vi "Distance Calc.vi"() -> ()   [LabVIEW 2014]
panel:
  out "Reference Distance \nin Inches":dbl
  out "Inch per \npixel Value":dbl
  out "Max Distance (Inches)":dbl
  out "Max Pixel Height":dbl
  out "Final Distance Array":dbl[](array[numeric])
  out "CM Heights Array":dbl[](array[numeric])
  in  "Particle Points":dbl[][](array[numeric])
  # "CM(X), CM(Y), Left X, Right X"
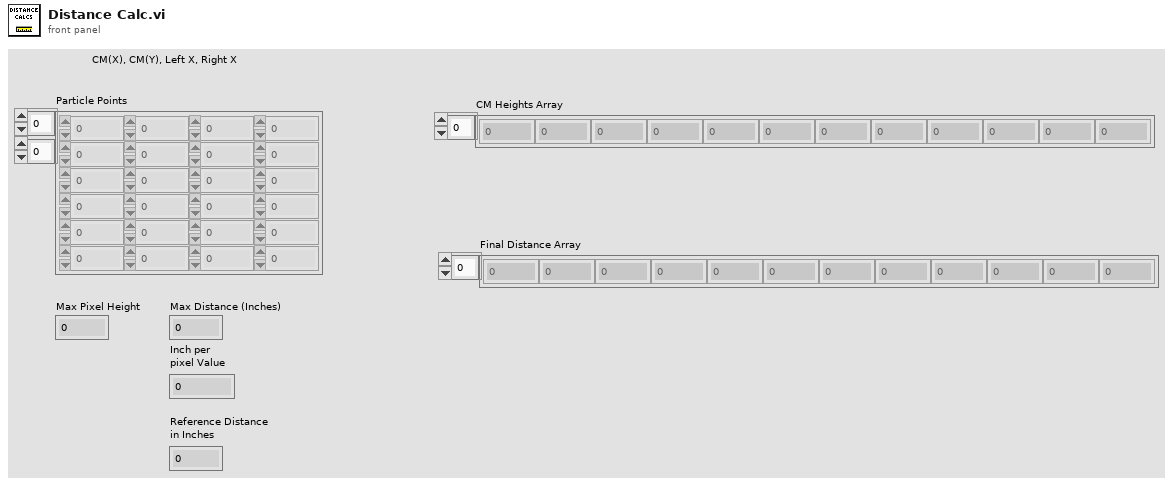
[diagram p1: front panel]
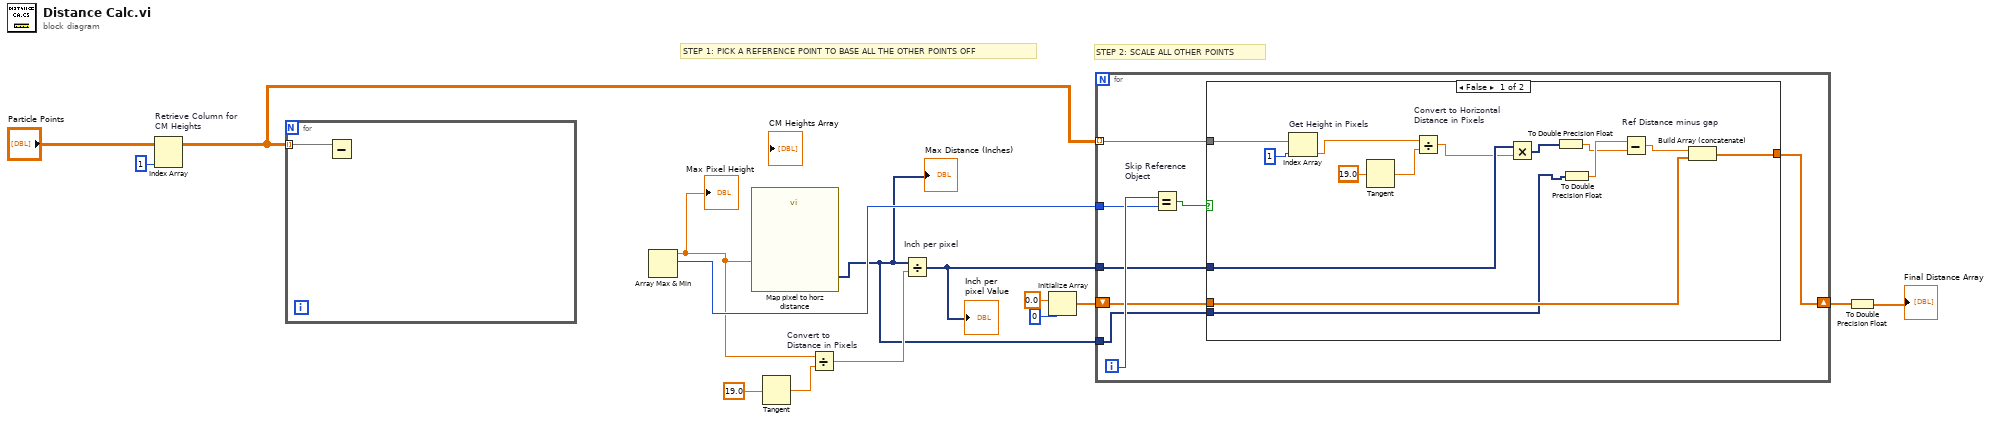
[diagram p0: block diagram]
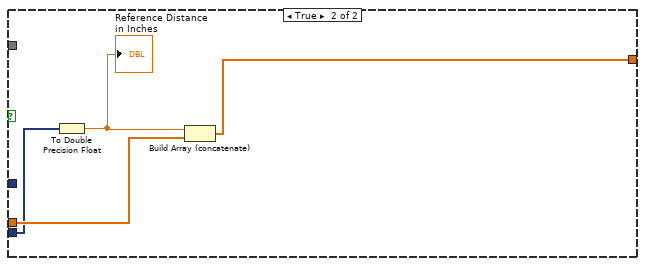
[diagram p2: hidden frame]
diagram:
  # "STEP 2: SCALE ALL OTHER POINTS"
  # "STEP 1: PICK A REFERENCE POINT TO BASE ALL THE OTHER POINTS OFF"
  n1 = Index Array "Retrieve Column for \nCM Heights"(array="Particle Points", index (col)=1 ("disabled index (col)")) -> ()  [unwired: 1 in, 1 out]
  n2 = for {
    tunnel: "Particle Points" -> [w15] mode=indexing
    n3 = Subtract(x=w15) -> ()  [unwired: 1 in, 1 out]
  }
  n4 = Array Max & Min() -> (max value=w10:dbl, max index (indices)=w13:i32)  [unwired: 1 in, 2 out]
  "Max Pixel Height" <- w10
  n5 = call "Map pixel to horz distance"("Signals"=w10) -> ("Scaled Signals"=w2:dynamicdata)  [unwired: 9 in, 1 out]
  "Max Distance (Inches)" <- w2
  n6 = Tangent(1:19.0 ("x")) -> (0:w11:dbl)
  n7 = Divide "Convert to \nDistance in Pixels"(x=w10, y=w11) -> (x/y=w9:dbl)
  n8 = Divide "Inch per pixel"(x=w2, y=w9) -> (x/y=w8:dynamicdata)
  "Inch per \npixel Value" <- w8
  n9 = Initialize Array(0.0 ("element"), 0 ("dimension size")) -> (w5:dbl[])
  n10 = for {
    tunnel: "Particle Points" -> [w23] mode=indexing
    tunnel: w13 -> [w21]
    tunnel: w8 -> [w19]
    shift-right: [w17] -> w7
    shift-left: w5 -> [w18]
    tunnel: w2 -> [w16]
    i -> [w22]
    n11 = Equal? "Skip Reference \nObject"(x=w22, y=w21) -> (x = y?=w20:bool)
    n12 = case shown="False" w20 {
      tunnel: w23 -> [w36 _]
      tunnel: w19 -> [w32 _]
      tunnel: w18 -> [w30 w41]
      tunnel: [w29 w40] -> w17
      tunnel: w16 -> [w27 w38]
      frame False {
        (unwired) 19.0 ("x")
        n13 = Index Array "Get Height in Pixels"(array=w36, index=1) -> (element=w34:dbl)
        n14 = Tangent(1:19.0 ("x")) -> (0:w33:dbl)
        n15 = Divide "Convert to Horizontal\nDistance in Pixels"(x=w34, y=w33) -> (x/y=w31:dbl)
        n16 = Multiply(x=w32, y=w31) -> (x*y=w28:dynamicdata)
        n17 = To Double Precision Float(number=w28) -> (double precision float=w25:dbl)
        n18 = To Double Precision Float(number=w27) -> (double precision float=w26:dbl)
        n19 = Subtract "Ref Distance minus gap"(x=w26, y=w25) -> (x-y=w24:dbl)
        n20 = Build Array (concatenate)(w24, w30) -> (w29:dbl[])
      }
      frame True {
        n21 = To Double Precision Float(number=w38) -> (double precision float=w39:dbl)
        "Reference Distance \nin Inches" <- w39
        n22 = Build Array (concatenate)(w39, w41) -> (w40:dbl[])
      }
    }
  }
  n23 = To Double Precision Float(number=w7) -> (double precision float=→"Final Distance Array":dbl[])
